vi "GetFrontPanel.vi"(8 "Error In":errorcluster, 11 "object in":refnum<class "Footer.lvclass">) -> (0 "Error Out":errorcluster, 2 "FrontPanel":refnum<class "FrontPanelControl.lvclass">, 3 "object out":refnum<class "Footer.lvclass">)   [LabVIEW 2021, in "Footer.lvclass"]
doc: "Retrieve the FrontPanelControl for controlling the state of the user interface front panel"
uses:
  Footer.lvclass
  .Externals/Library_UserInterface_FrontPanelControl/FrontPanelControl/FrontPanelControl.lvclass
  FooterGUI.vi
  Footer.lvclass/Footer.ctl
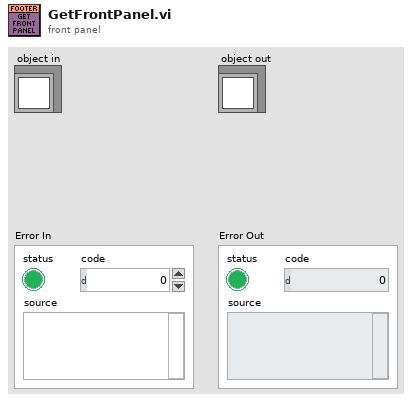
[diagram p1: front panel]
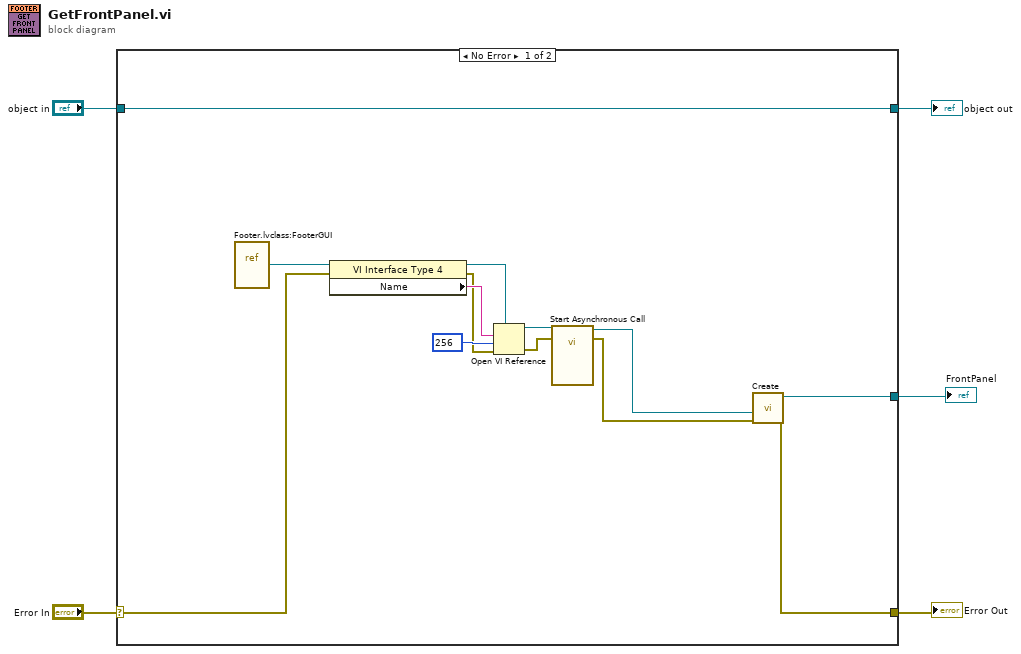
[diagram p0: block diagram]
diagram:
  n1 = case shown="No Error" "Error In" {
    selector: "Error In" -> [w7 w20]
    tunnel: [w11 w20] -> w4
    tunnel: [w18 w19] -> w2
    tunnel: "object in" -> [w18 w19]
    tunnel: [w6 _] -> w1
    frame No Error {
      n2 = vi-ref "Footer.lvclass:FooterGUI.vi"() -> (w17:refnum<vi>)
      n3 = property class="VI Interface Type 4"(reference=w17, error in=w7) -> (reference out=w16:refnum<vi>, error out=w8:errorcluster, "Name"=w15:string)
      n4 = Open VI Reference(type specifier VI Refnum (for type only)=w16, vi path=w15, options=256, error in (no error)=w8) -> (vi reference=w13:refnum<vi>, error out=w12:errorcluster)  [unwired: 2 in]
      n5 = call-by-ref "Start Asynchronous Call"(reference=w13, error in=w12) -> (reference out=w10:refnum<vi>, error out=w9:errorcluster)  [unwired: 12 in]
      n6 = call "Create.vi"("ErrorIn"=w9, "VIRef"=w10) -> ("ErrorOut"=w11:errorcluster, "ObjectOut"=w6:refnum<class "FrontPanelControl.lvclass">)  [unwired: 8 in]
    }
    frame Error {
    }
  }
  "Error Out" <- w4
  "object out" <- w2
  "FrontPanel" <- w1
